vi "2100_Test_Guardian Switch_No Publish Data_w_Config.vi"(0 "Semiconductor Module Context":T7, 1 "SMU Current Settings":T6={"OFF_Current  Range"=1e-05, "OFF_Current  Level"=-1e-05, "ON_Current  Range"=0.001, "ON_Current  Level"=0.001} {"ON_Current  Level" format="%#_6p"; "ON_Current  Range" format="%#_6p"; "OFF_Current  Level" format="%#_6p"; "OFF_Current  Range" format="%#_6p"}, 2 "Master_Register_Data_Array_In":T1 {"Address" format="%.0x"}, 5 "Script_Info":T3={"Script Name"="WalkingState", "All_Scripts"=[]}, 7 "Set_Meas_Sense":i32(ring)=1009 items=["Local"=1008, "Remote"=1009], 9 "USID":T4 max=15, 11 "Error In":errorcluster, 12 "Instrument_Pins":T5={"SMU_Pins"=["RF1", "RF2", "RF3", "RF4"], "HSDIO_Pins"=["CLK", "SDA"]}, 13 "Reg_Map_Bit_Name":string="RFC_SH", 14 "Reg_Map":string[][](array[string])=[["Reg Addr(0x00)", "7", "6", "5", "4", "3", "2", "1", "0"], ["0", "SPARE", "RF3_SH", "RF2_SH", "RF1_SH", "SPARE", "RF3_RFC", "RF2_RFC", "RF1_RFC"], ["1", "SPARE[7:0]", "", "", "", "", "", "", ""], ["2", "VVAR_EN", "LCM_EN", "RFC_SH", "SPARE", "VARACTOR[3:0]", "", "", ""], ["3", "SW_CTRL1_VIRTUAL[7:0]", "", "", "", "", "", "", ""], ["4", "SW_CTRL1_SWAP", "SW_CTRL1_RBSHIFT[2:0]", "", "", "SW_CTRL1_VSID[3:0]", "", "", ""], ["5", "REG_00_VIRTUAL_MASK[7:0]", "", "", "", "", "", "", ""], ["6", "LOCK_STATUS[1:0]", "", "CLK_DITHER", "FUSES_BURNED", "CLK_IDAC_CAL[3:0]", "", "", ""], ["7", "SPARE[2:0]", "", "", "ODFT_TRIM[4:0]", "", "", "", ""], ["8", "SPARE[2:0]", "", "", "HV_TRIM[4:0]", "", "", "", ""], ["9", "TEST_MUX[2:0]", "", "", "SPARE[1:0]", "", "MEMS_BG_TC[1:0]", "", "MEMSCP_RCM"], ["A", "CP_BOOST_OVRD_EN", "SPARE[2:0]", "", "", "PS_OFF_TIMER[1:0]", "", "PS_ON_TIMER[1:0]", ""], ["0", "", "", "", "", "", "", "", ""], ["D", "Reserved[1:0]", "", "WD_HI_EVENT_CNT[5:0]", "", "", "", "", ""], ["E", "VERSION_ID[7:0]", "", "", "", "", "", "", ""], ["F", "Reserved", "COUNT_200_LSB[6:0]", "", "", "", "", "", ""], ["10", "CLK_DIV2_EN", "Spare", "ODFT_EN", "HV_HYST[4:0]", "", "", "", ""], ["0", "", "", "", "", "", "", "", ""], ["12", "SHORT_FUSE", "FUSE_BURN", "STROBE_EN", "VIO_OK", "RTH[1:0]", "", "FUSE_LOAD_MAN_EN", "FUSE_LOAD"], ["13", "RR_ACK_EN", "Reserved", "ACK_POSITION[1:0]", "", "SuBUS_DRIVE_STRENGTH[3:0]", "", "", ""], ["14", "TM_IO_EN", "TM_IO_SEL", "SuBUS_OVS[1:0]", "", "Reserved[3:0]", "", "", ""], ["15", "Reserved[4:0]", "", "", "", "", "SuBUS_VERSION_PRESENT", "SuBUS_VOLTAGE", "SuBUS_FLAVOR_DEF"], ["16", "PROG_STROBE1_DUR[7:0]", "", "", "", "", "", "", ""], ["17", "PROG_STROBE0_DUR[7:0]", "", "", "", "", "", "", ""], ["18", "Reserved[2:0]", "", "", "EFUSE_SINGLE_ADDR_SEL[4:0]", "", "", "", ""], ["19", "POLL_ADR[4:0]", "", "", "", "", "POLL_BC[2:0]", "", ""], ["1A", "SOFTWARE_RESET", "Reserved[6:0]", "", "", "", "", "", ""], ["1B", "Reserved[7:0]", "", "", "", "", "", "", ""], ["1C", "PWR_MODE_1", "PWR_MODE_0", "TRIGGER_MASK[2:0]", "", "", "TRIGGER[2:0]", "", ""], ["1D", "PRODUCT_ID[7:0]", "", "", "", "", "", "", ""], ["1E", "MANUFACTURER_ID_LSB[7:0]", "", "", "", "", "", "", ""], ["1F", "MANUFACTURER_ID_MSB[3:0]", "", "", "", "USID[3:0]", "", "", ""]]) -> (6 "Master_Register_Data_Array_Out":T1 {"Address" format="%.0x"}, 8 "R_Guardian":dbl[](array[numeric]), 15 "Error Out":errorcluster)   [LabVIEW 2013]
uses:
  Controls/USID.ctl
  <vilib>/NI_TestStand_SemiconductorModule/NI_TestStand_Semiconductor_Module.lvlibp/PinMap/General/SemiconductorModuleContext.ctl
  Controls/Master_Reg_Data_Array.ctl
  Controls/Reg_Address_Data.ctl
  <vilib>/NI_TestStand_SemiconductorModule/NI_TestStand_Semiconductor_Module.lvlibp
panel:
  out "R Array":dbl[][](array[numeric])
  in  "Tab Control":enum32{"Test Info", "Instrument Settings"}(tab)
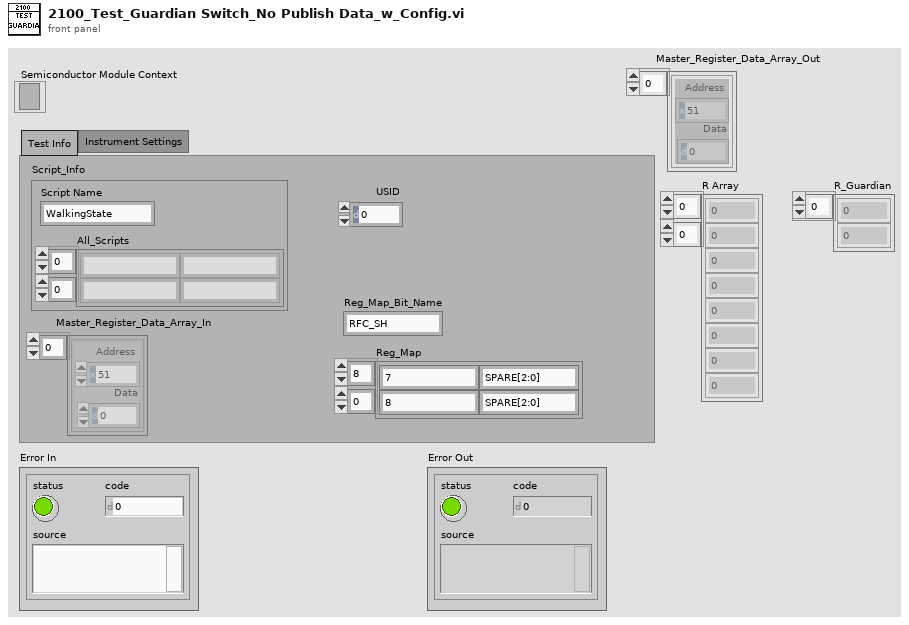
[diagram p1: front panel]
types:
  T1 = typedef "Master_Reg_Data_Array.ctl" = T2[]
  T2 = typedef "Reg_Address_Data.ctl" = cluster{"Address":u8, "Data":u8}
  T3 = cluster{"Script Name":string, "All_Scripts":string[][]}
  T4 = typedef "USID.ctl" = u8
  T5 = cluster{"SMU_Pins":string[], "HSDIO_Pins":string[]}
  T6 = cluster{"OFF_Current  Range":dbl, "OFF_Current  Level":dbl, "ON_Current  Range":dbl, "ON_Current  Level":dbl}
  T7 = typedef "NI_TestStand_Semiconductor_Module.lvlibp/SemiconductorModuleContext.ctl" = refnum<k7>
  T8 = typedef "Script Functions_Array.ctl" = enum16{"Reg_Write", "Bit_Write", "Delay", "Read", "Measure"}[]
  T9 = enum16{"Reg_Write", "Bit_Write", "Delay", "Read", "Measure"}
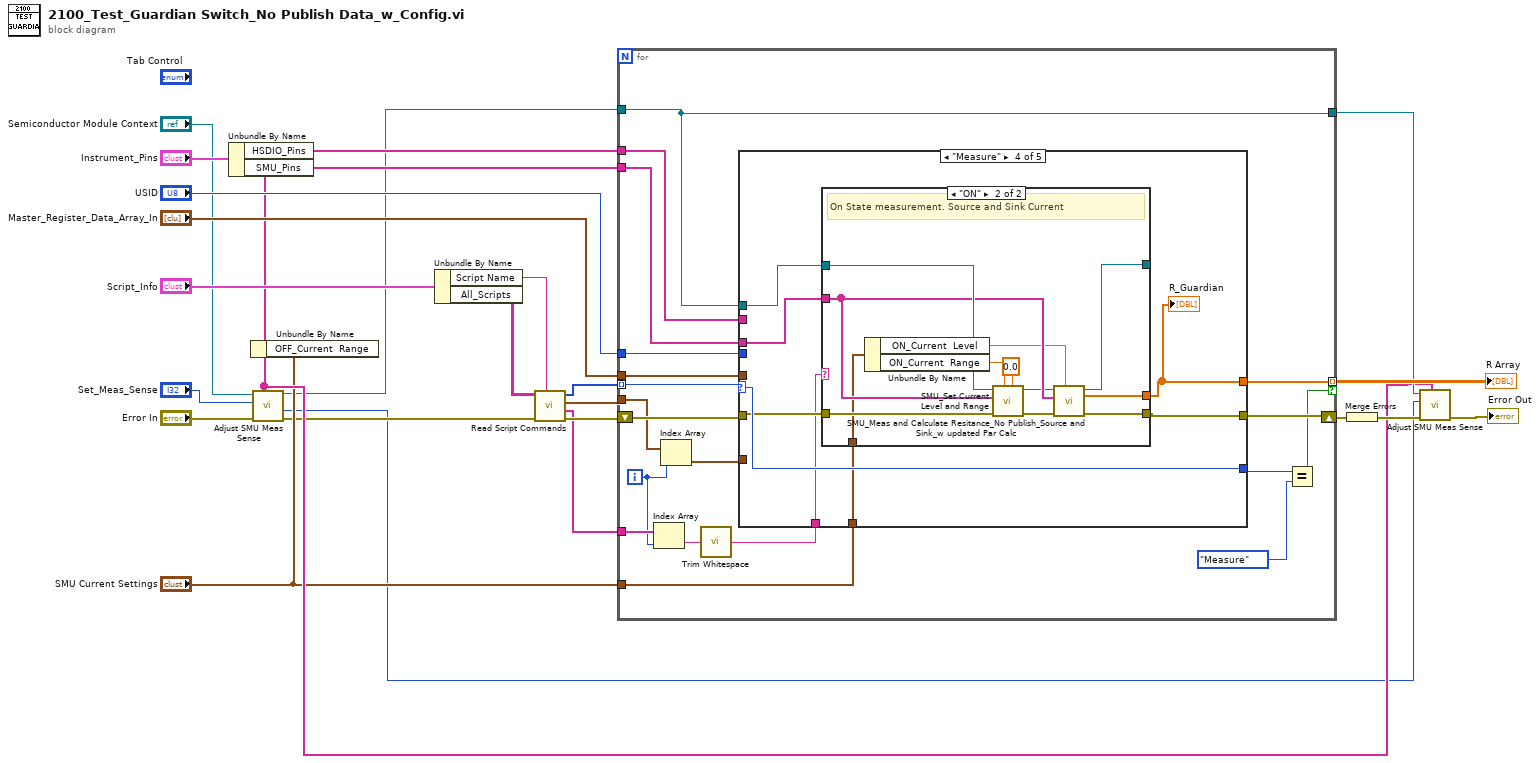
[diagram p0: block diagram]
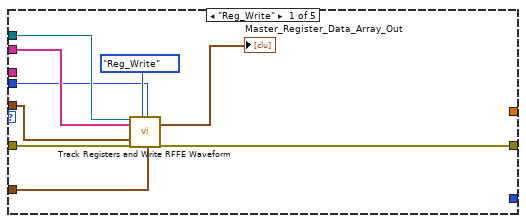
[diagram p2: hidden frame]
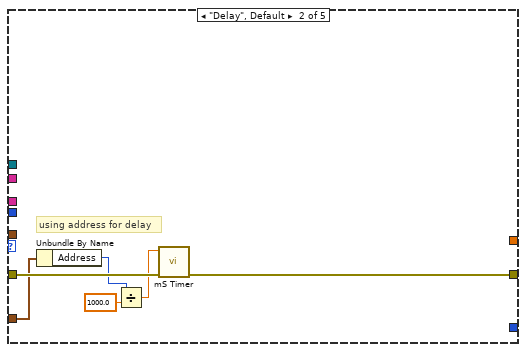
[diagram p3: hidden frame]
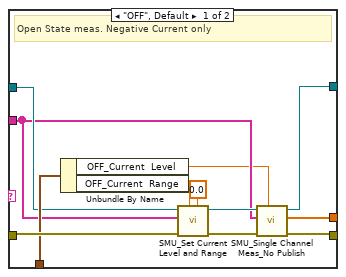
[diagram p5: hidden frame]
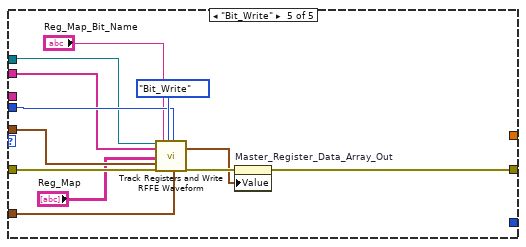
[diagram p6: hidden frame]
diagram:
  n1 = Unbundle By Name("Instrument_Pins") -> ("HSDIO_Pins"=w17:string[], "SMU_Pins"=w7:string[])
  n2 = Unbundle By Name("SMU Current Settings") -> ()  [unwired: 1 out]
  n3 = call "Adjust SMU Meas Sense.vi"("Pins"=w7, "error in (no error)"="Error In", "Set_Meas_Sense"="Set_Meas_Sense", "Semiconductor Module Context"="Semiconductor Module Context") -> ("error out"=w2:errorcluster, "Measurement:Sense"=w1:i32, "Semiconductor Module Context Out"=w3:T7)  [unwired: 5 in]
  n4 = Unbundle By Name("Script_Info") -> ("Script Name"=w14:string, "All_Scripts"=w15:string[][])
  n5 = call "Read Script Commands.vi"("Test Name"=w14, "Error In"=w2, "All_Scripts"=w15) -> ("Error Out"=w21:errorcluster, "Script_Note"=w6:string[], "Script_Data"=w22:T2[], "Script_Functions"=w23:T8)  [unwired: 5 in]
  n6 = for {
    tunnel: "USID" -> [w38]
    tunnel: w23 -> [w37] mode=indexing
    tunnel: w22 -> [w41]
    tunnel: w3 -> [w30]
    tunnel: w17 -> [w42]
    shift-right: [w36] -> w19
    shift-left: w21 -> [w43]
    tunnel: "Master_Register_Data_Array_In" -> [w39]
    tunnel: w7 -> [w35]
    tunnel: [w31] -> w13 mode=indexing if=w32
    tunnel: [w30] -> w8
    tunnel: "SMU Current Settings" -> [w29]
    tunnel: w6 -> [w27]
    i -> [w26]
    n7 = Index Array(array=w27, index=w26) -> (element=w28:string)
    n8 = Index Array(array=w41, index=w26) -> (element=w40:T2)
    n9 = call <vilib>:"Trim Whitespace.vi"("string"=w28) -> ("trimmed string"=w25:string)  [unwired: 1 in]
    n10 = case shown="\"Measure\"" w37 {
      selector: w37 -> [_ _ _ w67 _]
      tunnel: w40 -> [w47 w57 _ _ w96]
      tunnel: w43 -> [w52 w58 w59 w66 w103]
      tunnel: w38 -> [w44 _ _ _ w101]
      tunnel: w30 -> [w50 _ _ w63 w100]
      tunnel: w42 -> [w49 _ _ _ w99]
      tunnel: [w51 w56 w59 w65 w93] -> w36
      tunnel: w39 -> [w46 _ _ _ w97]
      tunnel: w35 -> [_ _ _ w62 _]
      tunnel: [_ _ _ w67 _] -> w34
      tunnel: [_ _ _ w64 _] -> w31
      tunnel: w29 -> [_ _ _ w60 _]
      tunnel: w25 -> [_ _ _ w61 _]
      frame "Reg_Write" {
        n11 = call "Track Registers and Write RFFE Waveform.vi"("Semiconductor Module Context"=w50, "Pins"=w49, "Master_Register_Data_Array_In"=w46, "Error In"=w52, "Script_Functions"=enum16{"Reg_Write", "Bit_Write"}."Reg_Write", "USID"=w44, "Reg_Address_Data"=w47) -> ("Master_Register_Data_Array_Out"=→"Master_Register_Data_Array_Out":T1, "Error Out"=w51:errorcluster)  [unwired: 10 in, 1 out]
      }
      frame "Delay", Default {
        # "using address for delay"
        n12 = Unbundle By Name(w57) -> ("Address"=w54:u8)
        n13 = Divide(x=w54, y=1000.0) -> (x/y=w53:dbl)
        n14 = call "mS Timer.vi"("Error In"=w58, "Delay(S)"=w53) -> ("Error Out"=w56:errorcluster)  [unwired: 9 in]
      }
      frame "Read" {
      }
      frame "Measure" {
        n15 = case shown="\"ON\"" w61 {
          tunnel: w66 -> [w76 w90]
          tunnel: w60 -> [w75 w83]
          tunnel: w63 -> [w74 w86]
          tunnel: [w73 w88] -> _
          tunnel: w62 -> [w72 w85]
          tunnel: [w70 w87] -> w64
          tunnel: [w69 w89] -> w65
          frame "OFF", Default {
            # "Open State meas. Negative Current only"
            n16 = Unbundle By Name(w75) -> ("OFF_Current  Level"=w71:dbl, "OFF_Current  Range"=w79:dbl)
            n17 = call "SMU_Set Current Level and Range.vi"("current level"=0.0, "current range"=w79, "error in (no error)"=w76, "Pins"=w72, "Semiconductor Module Context"=w74) -> ("error out"=w78:errorcluster, "Semiconductor Module Context Out"=w77:T7)  [unwired: 5 in]
            n18 = call "SMU_Single Channel Meas_No Publish.vi"("Meas_A_Level"=w71, "error in (no error)"=w78, "Pins"=w72, "Semiconductor Module Context"=w77) -> ("error Out"=w69:errorcluster, "R Array"=w70:dbl[], "Semiconductor Module Context Out"=w73:T7)  [unwired: 5 in]
          }
          frame "ON" {
            # "On State measurement. Source and Sink Current"
            n19 = Unbundle By Name(w83) -> ("ON_Current  Level"=w81:dbl, "ON_Current  Range"=w82:dbl)
            n20 = call "SMU_Set Current Level and Range.vi"("current level"=0.0, "current range"=w82, "error in (no error)"=w90, "Pins"=w85, "Semiconductor Module Context"=w86) -> ("error out"=w91:errorcluster, "Semiconductor Module Context Out"=w84:T7)  [unwired: 5 in]
            n21 = call "SMU_Meas and Calculate Resitance_No Publish_Source and Sink_w updated Par Calc.vi"("Current  Level"=w81, "error in (no error)"=w91, "Pins"=w85, "Semiconductor Module Context"=w84) -> ("error Out"=w89:errorcluster, "R Array"=w87:dbl[], "Semiconductor Module Context Out"=w88:T7)  [unwired: 4 in, 1 out]
          }
        }
        "R_Guardian" <- w64
      }
      frame "Bit_Write" {
        n22 = call "Track Registers and Write RFFE Waveform.vi"("Semiconductor Module Context"=w100, "Pins"=w99, "Reg_Map"="Reg_Map", "Master_Register_Data_Array_In"=w97, "Error In"=w103, "Reg_Map_Bit_Name"="Reg_Map_Bit_Name", "Script_Functions"=enum16{"Reg_Write", "Bit_Write"}."Bit_Write", "USID"=w101, "Reg_Address_Data"=w96) -> ("Master_Register_Data_Array_Out"=w92:T1, "Error Out"=w94:errorcluster)  [unwired: 8 in, 1 out]
        n23 = property on="Master_Register_Data_Array_Out" class="Arr (strict)"(error in=w94, "Value"=w92) -> (error out=w93:errorcluster)  [unwired: 1 in, 1 out]
      }
    }
    n24 = Equal?(x=w34, y=T9."Measure" ("Enum")) -> (x = y?=w32:bool)
  }
  "R Array" <- w13
  n25 = Merge Errors(w19) -> (w10:errorcluster)
  n26 = call "Adjust SMU Meas Sense.vi"("Pins"=w7, "error in (no error)"=w10, "Set_Meas_Sense"=w1, "Semiconductor Module Context"=w8) -> ("error out"=→"Error Out":errorcluster)  [unwired: 5 in, 2 out]
